vi "main.vi"() -> ()   [LabVIEW 2022 SP3]
uses:
  <vilib>/sound2/lvsound2.llb/Sampling Mode.ctl
  <vilib>/sound2/lvsound2.llb/Sound File Position.ctl
  <vilib>/sound2/lvsound2.llb/Sound File Read Open.vi
  <vilib>/sound2/lvsound2.llb/Sound File Info (refnum).vi
  <vilib>/sound2/lvsound2.llb/Sound File Read (DBL).vi
  <vilib>/sound2/lvsound2.llb/Sound Output Write (DBL).vi
panel:
  in  "stop":bool
  out "x+y":dbl
  in  "device ID":u32
  in  "Path":path
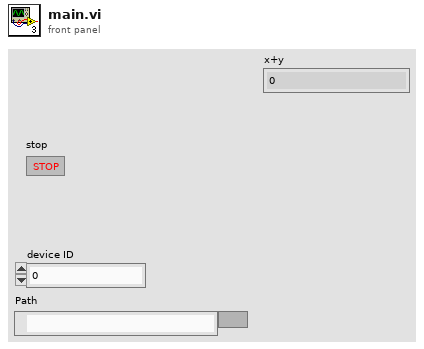
[diagram p1: front panel]
types:
  T1 = typedef "Sampling Mode.ctl" = i32
  T2 = typedef "Sound File Refnum.ctl" = refnum<file>
  T3 = typedef "Sound Data Format.ctl" = cluster{"sample rate (S/s)":dbl, "number of channels":i32, "bits per sample":i32}
  T4 = typedef "Sound Output Task ID.ctl" = u32
  T5 = typedef "Sound File Position.ctl" = u16
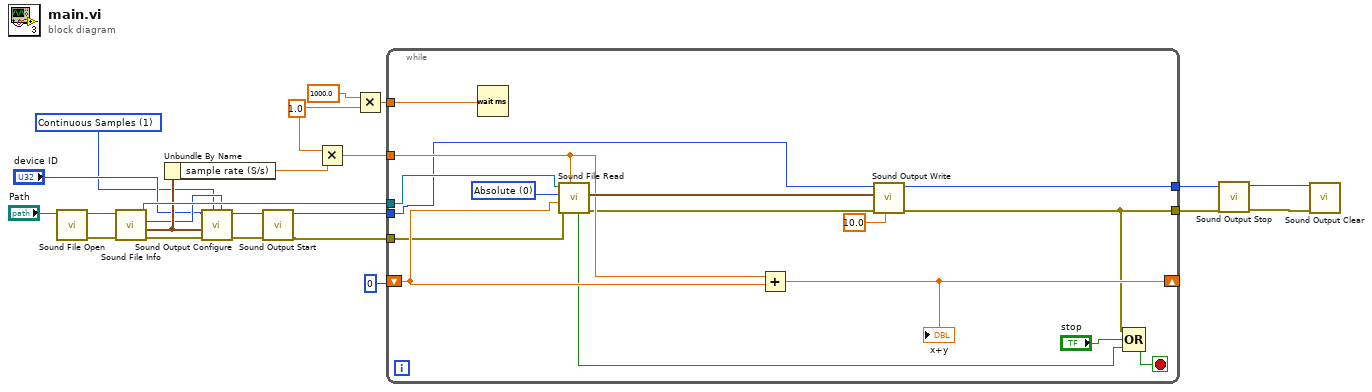
[diagram p0: block diagram]
diagram:
  w11 = 1.0 ("period")
  w1 = T1 1 items=["Finite Samples", "Continuous Samples"] ("sample mode")
  n1 = call-poly <vilib>:"Sound File Open.vi"("path"="Path") -> ("error out"=w21:errorcluster, "sound file refnum"=w22:T2)  [unwired: 9 in]
  n2 = call-poly <vilib>:"Sound File Info.vi"("error in (no error)"=w21, "sound file refnum"=w22) -> ("error out"=w8:errorcluster, "sound format"=w7:T3, "total number of samples/ch"=w3:u32, "sound file refnum out"=w20:T2)  [unwired: 6 in]
  n3 = Unbundle By Name(w7) -> ("sample rate (S/s)"=w4:dbl)
  n4 = call <vilib>:"Sound Output Configure.vi"("number of samples/ch"=w3, "sample mode"=w1, "error in (no error)"=w8, "sound format"=w7, "device ID"="device ID") -> ("error out"=w9:errorcluster, "task ID"=w10:T4)  [unwired: 5 in]
  n5 = call <vilib>:"Sound Output Start.vi"("error in (no error)"=w9, "task ID"=w10) -> ("error out"=w6:errorcluster, "task ID out"=w5:T4)  [unwired: 8 in]
  n6 = Multiply(x=w11, y=w4) -> (x*y=w14:dbl)
  n7 = Multiply(x=1000.0, y=w11) -> (x*y=w12:dbl)
  n8 = while {
    tunnel: [w25] -> w16
    tunnel: [w33] -> w18
    shift-right: [w36] -> _
    shift-left: 0 -> [w34]
    tunnel: w20 -> [w35]
    tunnel: w14 -> [w32]
    tunnel: w12 -> [w31]
    tunnel: w6 -> [w30]
    tunnel: w5 -> [w28]
    stop <- w24 stop-if-true
    w38 = T5 0 items=["Absolute"=0, "Relative"=2] ("position mode")
    n9 = Wait (ms)(milliseconds to wait=w31) -> ()  [unwired: 1 out]
    n10 = call-poly <vilib>:"Sound File Read.vi"("number of samples/ch (-1: all)"=w32, "error in (no error)"=w30, "position offset"=w34, "position mode"=w38, "sound file refnum"=w35) -> ("error out"=w29:errorcluster, "data"=w37:waveform(dbl)[], "end of file?"=w27:bool)  [unwired: 2 in, 2 out]
    n11 = Add(x=w32, y=w34) -> (x+y=w36:dbl)
    "x+y" <- w36
    n12 = call-poly <vilib>:"Sound Output Write.vi"("timeout (sec)"=10.0, "error in (no error)"=w29, "data"=w37, "task ID"=w28) -> ("error out"=w25:errorcluster, "task ID out"=w33:T4)  [unwired: 6 in]
    n13 = Compound Arithmetic op=OR(w25, "stop", w27) -> (w24:bool)
  }
  n14 = call <vilib>:"Sound Output Stop.vi"("error in (no error)"=w16, "task ID"=w18) -> ("error out"=w15:errorcluster, "task ID out"=w17:T4)  [unwired: 8 in]
  n15 = call <vilib>:"Sound Output Clear.vi"("error in (no error)"=w15, "task ID"=w17) -> ()  [unwired: 9 in, 1 out]
